vi "Create Winch Constants.vi"(1 "error in":errorcluster, 2 "localConstantSpreadSheet":string[][](array[string]), 3 "robotID":string) -> (0 "error out":errorcluster)   [LabVIEW 2020]
uses:
  2022 Robot Global Data.vi
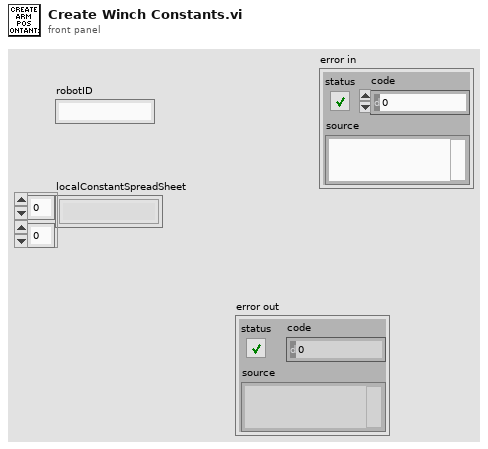
[diagram p1: front panel]
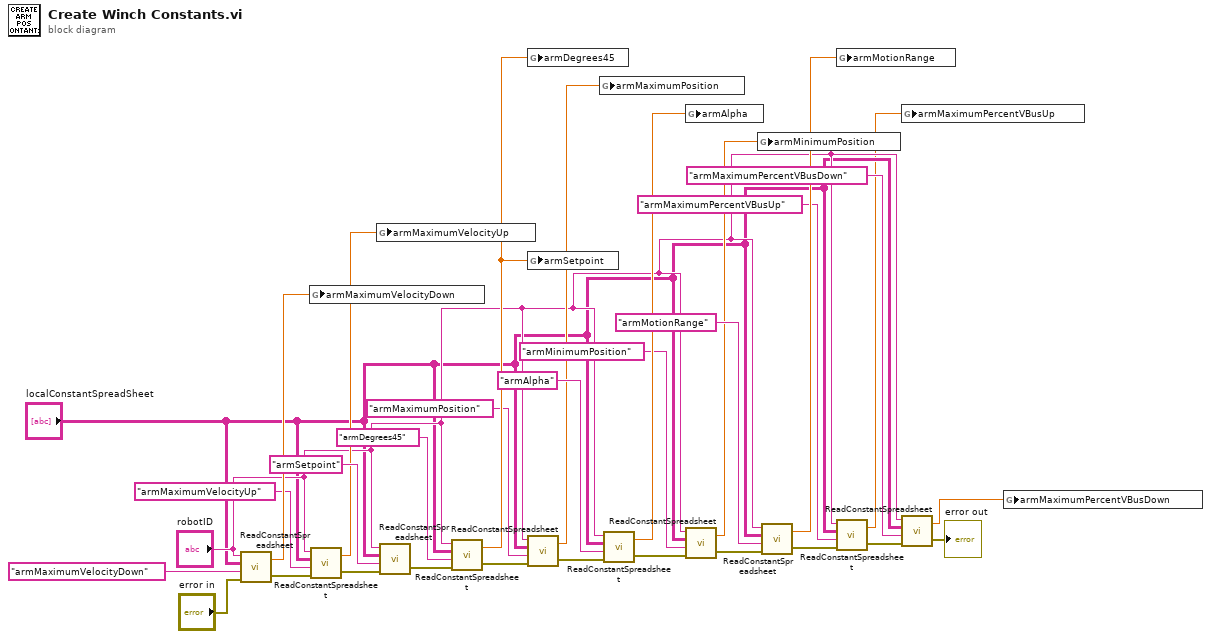
[diagram p0: block diagram]
diagram:
  n1 = call "ReadConstantSpreadsheet.vi"("error in"="error in", "Constant"="armMaximumVelocityDown", "2022ConstantSpreadSheet"="localConstantSpreadSheet", "Robot ID"="robotID") -> ("error out"=w9:errorcluster, "Constant Value"=w29:dbl)
  n2 = global write "2022 Robot Global Data.vi" "armMaximumVelocityDown"(w29) -> ()
  n3 = call "ReadConstantSpreadsheet.vi"("error in"=w9, "Constant"="armMaximumVelocityUp", "2022ConstantSpreadSheet"="localConstantSpreadSheet", "Robot ID"="robotID") -> ("error out"=w8:errorcluster, "Constant Value"=w7:dbl)
  n4 = global write "2022 Robot Global Data.vi" "armMaximumVelocityUp"(w7) -> ()
  n5 = call "ReadConstantSpreadsheet.vi"("error in"=w8, "Constant"="armSetpoint", "2022ConstantSpreadSheet"="localConstantSpreadSheet", "Robot ID"="robotID") -> ("error out"=w18:errorcluster)  [unwired: 1 out]
  n6 = call "ReadConstantSpreadsheet.vi"("error in"=w18, "Constant"="armDegrees45", "2022ConstantSpreadSheet"="localConstantSpreadSheet", "Robot ID"="robotID") -> ("error out"=w17:errorcluster, "Constant Value"=w31:dbl)
  n7 = global write "2022 Robot Global Data.vi" "armDegrees45"(w31) -> ()
  n8 = global write "2022 Robot Global Data.vi" "armSetpoint"(w31) -> ()
  n9 = call "ReadConstantSpreadsheet.vi"("error in"=w17, "Constant"="armMaximumPosition", "2022ConstantSpreadSheet"="localConstantSpreadSheet", "Robot ID"="robotID") -> ("error out"=w16:errorcluster, "Constant Value"=w24:dbl)
  n10 = global write "2022 Robot Global Data.vi" "armMaximumPosition"(w24) -> ()
  n11 = call "ReadConstantSpreadsheet.vi"("error in"=w16, "Constant"="armAlpha", "2022ConstantSpreadSheet"="localConstantSpreadSheet", "Robot ID"="robotID") -> ("error out"=w15:errorcluster, "Constant Value"=w27:dbl)
  n12 = global write "2022 Robot Global Data.vi" "armAlpha"(w27) -> ()
  n13 = call "ReadConstantSpreadsheet.vi"("error in"=w15, "Constant"="armMinimumPosition", "2022ConstantSpreadSheet"="localConstantSpreadSheet", "Robot ID"="robotID") -> ("error out"=w14:errorcluster, "Constant Value"=w23:dbl)
  n14 = global write "2022 Robot Global Data.vi" "armMinimumPosition"(w23) -> ()
  n15 = call "ReadConstantSpreadsheet.vi"("error in"=w14, "Constant"="armMotionRange", "2022ConstantSpreadSheet"="localConstantSpreadSheet", "Robot ID"="robotID") -> ("error out"=w6:errorcluster, "Constant Value"=w32:dbl)
  n16 = global write "2022 Robot Global Data.vi" "armMotionRange"(w32) -> ()
  n17 = call "ReadConstantSpreadsheet.vi"("error in"=w6, "Constant"="armMaximumPercentVBusUp", "2022ConstantSpreadSheet"="localConstantSpreadSheet", "Robot ID"="robotID") -> ("error out"=w5:errorcluster, "Constant Value"=w1:dbl)
  n18 = global write "2022 Robot Global Data.vi" "armMaximumPercentVBusUp"(w1) -> ()
  n19 = call "ReadConstantSpreadsheet.vi"("error in"=w5, "Constant"="armMaximumPercentVBusDown", "2022ConstantSpreadSheet"="localConstantSpreadSheet", "Robot ID"="robotID") -> ("error out"=→"error out":errorcluster, "Constant Value"=w13:dbl)
  n20 = global write "2022 Robot Global Data.vi" "armMaximumPercentVBusDown"(w13) -> ()
